vi "Parse_NaN.vi"(9 "values":dbl[](array[numeric]), 11 "timestamps_ns":u64[](array[numeric])) -> (1 "Filtered Values":dbl[](array[numeric]), 3 "Filtered Timestamps":u64[](array[numeric]))   [LabVIEW 2020, in "Nominal Streaming.lvlib" / "Channel.lvclass"]
uses:
  Channel.lvclass
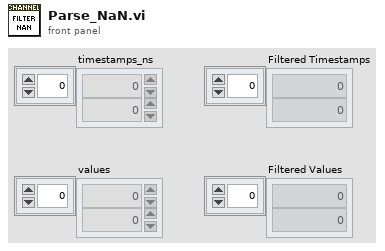
[diagram p1: front panel]
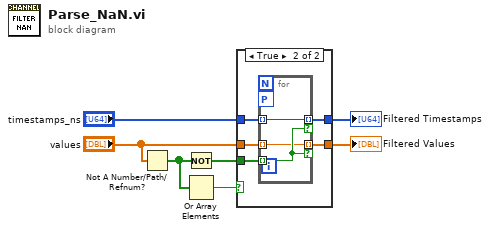
[diagram p0: block diagram]
diagram:
  n1 = Not A Number/Path/Refnum?(number/path/refnum="values") -> (NaN/Path/Refnum?=w5:bool[])
  n2 = Not(x=w5) -> (.not. x?=w7:bool[])
  n3 = Or Array Elements(Boolean array=w5) -> (logical OR=w6:bool)
  n4 = case shown="True" w6 {
    tunnel: w7 -> [_ w14]
    tunnel: "timestamps_ns" -> [w9 w13]
    tunnel: "values" -> [w8 w12]
    tunnel: [w9 w11] -> w4
    tunnel: [w8 w10] -> w3
    frame False {
    }
    frame True {
      n5 = for {
        tunnel: [w16] -> w11 mode=indexing if=w17
        tunnel: [w15] -> w10 mode=indexing if=w17
        tunnel: w14 -> [w17] mode=indexing
        workers-P: _ -> [_]
        tunnel: w13 -> [w16] mode=indexing
        tunnel: w12 -> [w15] mode=indexing
      }
    }
  }
  "Filtered Timestamps" <- w4
  "Filtered Values" <- w3
